vi "Update Status.vi"(9 "ID":i32, 10 "MyPosition":cluster{"X":i32, "Y":i32}, 11 "Mother in":refnum<class "Formics.lvclass">) -> (3 "Mother out":refnum<class "Formics.lvclass">)   [LabVIEW 2015, in "Formics.lvclass"]
uses:
  Formics.lvclass
  Formics.lvclass/Formics.ctl
  SquareStatus.ctl
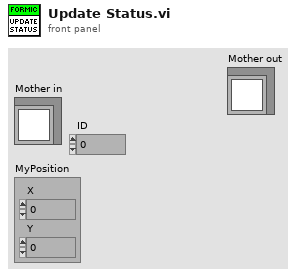
[diagram p1: front panel]
types:
  T1 = typedef "Formics.lvclass/SquareStatus DVR.ctl" = refnum<data-value>
  T2 = typedef "Formics.lvclass/SquareStatus.ctl" = cluster{"ID":i32, "Heartbeat":bool, "MyPosition":cluster{"X":i32, "Y":i32}}
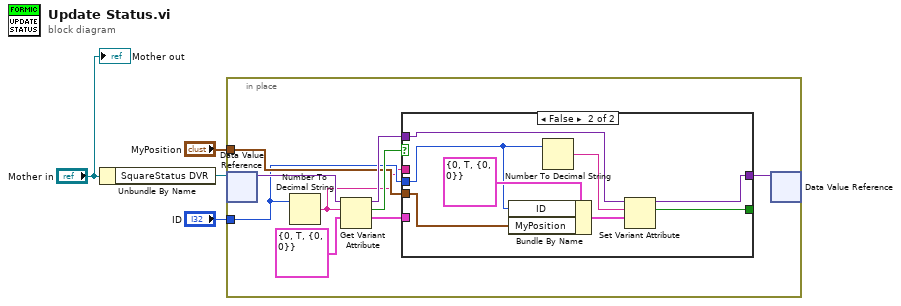
[diagram p0: block diagram]
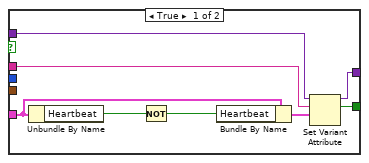
[diagram p2: hidden frame]
diagram:
  n1 = Unbundle By Name("Mother in") -> ("SquareStatus DVR"=w3:T1)
  n2 = in-place {
    in-place-border: "MyPosition" -> [w7]
    in-place-border: "ID" -> [w6]
    n3 = in-place-dvr #1(w3) -> (w12:variant)  [unwired: 1 out]
    n4 = Number To Decimal String(number=w6) -> (decimal integer string=w5:string)  [unwired: 1 in]
    n5 = Get Variant Attribute(Variant=w12, name=w5, default value (empty Variant)=T2 {"ID"=0, "Heartbeat"=TRUE, "MyPosition"={"X"=0, "Y"=0}} ("Shared Info")) -> (duplicate Variant=w11:variant, found=w9:bool, value=w8:T2)  [unwired: 1 in, 1 out]
    n6 = case shown="False" w9 {
      tunnel: [w21 w29] -> w10
      tunnel: [w20 w28] -> _
      tunnel: w11 -> [w17 w27]
      tunnel: w8 -> [w15 _]
      tunnel: w5 -> [w14 _]
      tunnel: w7 -> [_ w23]
      tunnel: w6 -> [_ w22]
      frame True {
        n7 = Unbundle By Name(w15) -> ("Heartbeat"=w19:bool)
        n8 = Not(x=w19) -> (.not. x?=w18:bool)
        n9 = Bundle By Name(cluster=w15, "Heartbeat"=w18) -> (w16:T2)
        n10 = Set Variant Attribute(Variant=w17, name=w14, value=w16) -> (Variant out=w21:variant, replaced=w20:bool)  [unwired: 1 in, 1 out]
      }
      frame False {
        n11 = Bundle By Name(cluster=T2 {"ID"=0, "Heartbeat"=TRUE, "MyPosition"={"X"=0, "Y"=0}} ("Shared Info"), "ID"=w22, "MyPosition"=w23) -> (w25:T2)
        n12 = Number To Decimal String(number=w22) -> (decimal integer string=w24:string)  [unwired: 1 in]
        n13 = Set Variant Attribute(Variant=w27, name=w24, value=w25) -> (Variant out=w29:variant, replaced=w28:bool)  [unwired: 1 in, 1 out]
      }
    }
    n14 = in-place-dvr #1(w10) -> ()  [unwired: 2 out]
  }
  "Mother out" <- "Mother in"
